vi "Apply Pump Turbine Scaling.vi"(1 "EtherCAT System State IN":map{string, dbl}(c390)) -> (0 "EtherCAT System State OUT":map{string, dbl}(c390))   [LabVIEW 2024, in "Hardware Controller.lvlib"]
uses:
  Hardware Controller.lvlib
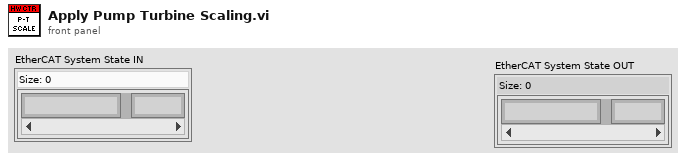
[diagram p1: front panel]
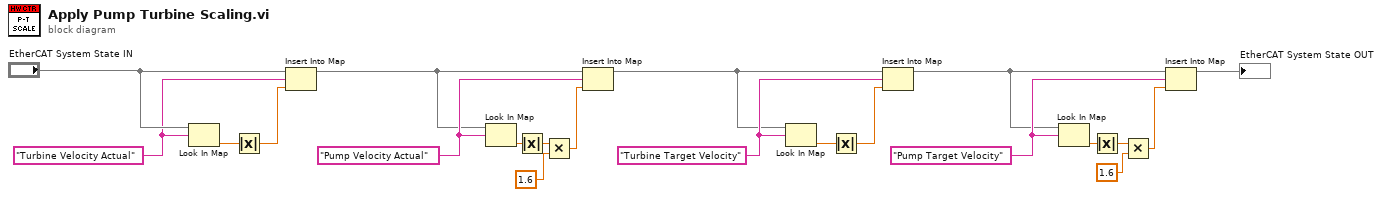
[diagram p0: block diagram]
diagram:
  w7 = "Pump Target Velocity"
  w13 = "Turbine Target Velocity"
  w17 = "Pump Velocity Actual"
  w20 = "Turbine Velocity Actual"
  n1 = Look In Map(map="EtherCAT System State IN", key=w20) -> (value=w19:dbl)  [unwired: 1 in, 1 out]
  n2 = Absolute Value(x=w19) -> (abs(x)=w18:dbl)
  n3 = Insert Into Map(map in="EtherCAT System State IN", key=w20, value=w18) -> (map out=w14:map{string, dbl})  [unwired: 2 out]
  n4 = Look In Map(map=w14, key=w17) -> (value=w16:dbl)  [unwired: 1 in, 1 out]
  n5 = Absolute Value(x=w16) -> (abs(x)=w15:dbl)
  n6 = Multiply(x=w15, y=1.6) -> (x*y=w5:dbl)
  n7 = Insert Into Map(map in=w14, key=w17, value=w5) -> (map out=w10:map{string, dbl})  [unwired: 2 out]
  n8 = Look In Map(map=w10, key=w13) -> (value=w12:dbl)  [unwired: 1 in, 1 out]
  n9 = Absolute Value(x=w12) -> (abs(x)=w11:dbl)
  n10 = Insert Into Map(map in=w10, key=w13, value=w11) -> (map out=w6:map{string, dbl})  [unwired: 2 out]
  n11 = Look In Map(map=w6, key=w7) -> (value=w8:dbl)  [unwired: 1 in, 1 out]
  n12 = Absolute Value(x=w8) -> (abs(x)=w9:dbl)
  n13 = Multiply(x=w9, y=1.6) -> (x*y=w3:dbl)
  n14 = Insert Into Map(map in=w6, key=w7, value=w3) -> (map out=→"EtherCAT System State OUT":map{string, dbl})  [unwired: 2 out]
